vi "Example 05a - Simple Arrays.vi"() -> ()   [LabVIEW 2020]
uses:
  Lua for LabVIEW/Lua/Lua.lvclass
panel:
  out "#x":dbl
  out "x":dbl[](array[numeric])
  out "error out":errorcluster
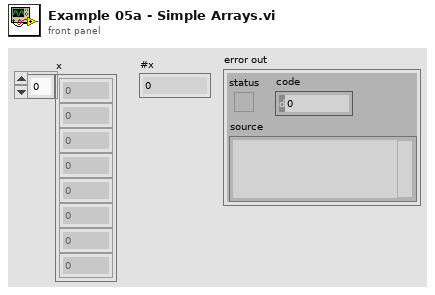
[diagram p1: front panel]
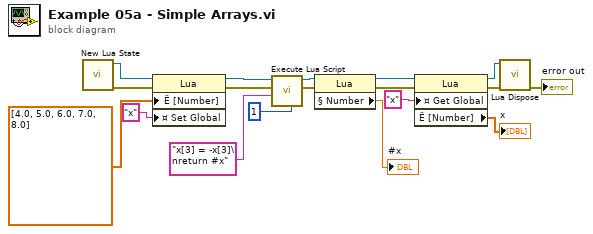
[diagram p0: block diagram]
diagram:
  n1 = call "New Lua State.vi"() -> ("error out"=w18:errorcluster, "Lua out"=w14:refnum<class "Lua.lvclass">)  [unwired: 10 in]
  n2 = property class="Lua"(reference=w14, error in=w18, "Ё [Number]"=dbl[] [4.0, 5.0, 6.0, 7.0, 8.0] ("§ [Number]"), "¤ Set Global"="x" ("(State) Get Global")) -> (reference out=w11:refnum<class "Lua.lvclass">, error out=w3:errorcluster)
  n3 = call-dynamic "Execute Lua Script.vi"("nresults"=1, "lua script"="x[3] = -x[3]\nreturn #x", "error in (no error)"=w3, "Lua in"=w11) -> ("error out"=w1:errorcluster, "Lua out"=w9:refnum<class "Lua.lvclass">)  [unwired: 6 in]
  n4 = property class="Lua"(reference=w9, error in=w1) -> (reference out=w8:refnum<class "Lua.lvclass">, error out=w7:errorcluster, "§ Number"=→"#x":dbl)
  n5 = property class="Lua"(reference=w8, error in=w7, "¤ Get Global"="x" ("(State) Get Global")) -> (reference out=w17:refnum<class "Lua.lvclass">, error out=w16:errorcluster, "Ё [Number]"=→"x":dbl[])
  n6 = call-dynamic "Lua Dispose.vi"("error in (no error)"=w16, "Lua in"=w17) -> ("error out"=→"error out":errorcluster)  [unwired: 9 in]
